vi "subStepper Motor.vi"(8 "error in":errorcluster, 9 "# of Pellet":dbl, 10 "Numeric":dbl, 11 "Arduino Resource":T1={"VISA resource"="", "Board Type"=enum."Uno", "Connection Type"=enum."USB / Serial", "Bytes Per Packet (15)"=15}) -> (0 "error out":errorcluster, 2 "Stepper Step":i32, 3 "Arduino Resource 2":T1={"VISA resource"="", "Board Type"=enum."Uno", "Connection Type"=enum."USB / Serial", "Bytes Per Packet (15)"=15})   [LabVIEW 2016]
uses:
  <vilib>/LabVIEW Interface for Arduino/Type Defs/Arduino Resource.ctl
  <vilib>/LabVIEW Interface for Arduino/Type Defs/Board Type.ctl
  <vilib>/LabVIEW Interface for Arduino/LabVIEW Interface for Arduino.lvlib
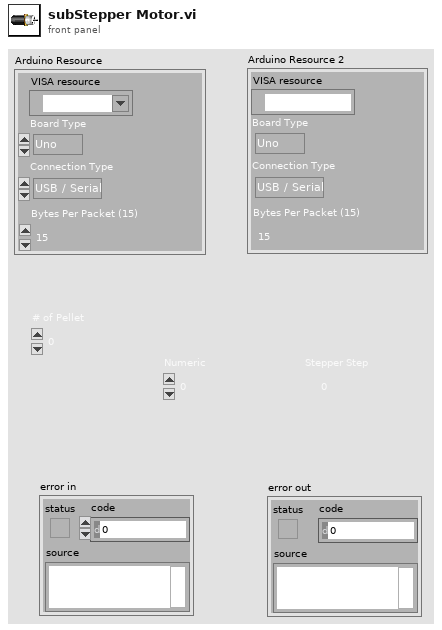
[diagram p1: front panel]
types:
  T1 = typedef "LabVIEW Interface for Arduino.lvlib/Arduino Resource.ctl" = cluster{"VISA resource":refnum<visa-resource-name>, "Board Type":T2, "Connection Type":enum8{"USB / Serial"}, "Bytes Per Packet (15)":u8}
  T2 = typedef "LabVIEW Interface for Arduino.lvlib/Board Type.ctl" = enum16{"Uno", "Dimuelanove w/Atmega 328", "Mega 2560"}
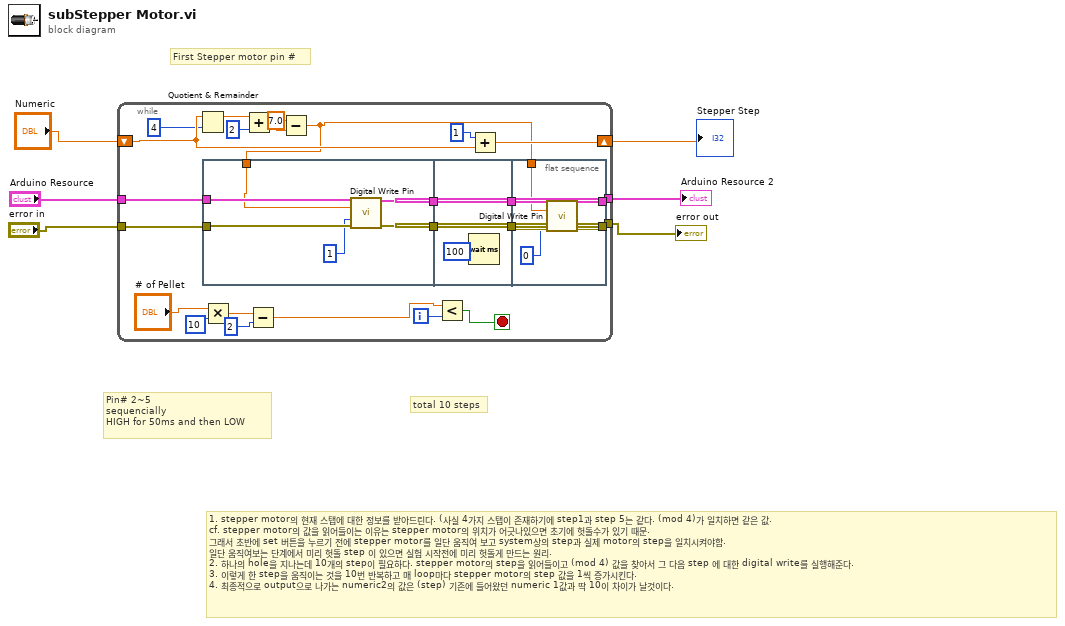
[diagram p0: block diagram]
diagram:
  # "1. stepper motor의 현재 스탭에 대한 정보를 받아드린다. (사실 4가지 스탭이 존재하기에 step1과 step 5는 같다. (mod 4)가 일치하면 같은 값.\ncf. stepper motor의 값을 읽어들이는 이유는 stepper motor의 위치가 어긋나있으면 초기에 헛돌수가 있기 때문. \n그래서 초반에 set 버튼을 누르기 전에 stepper motor를 일단 움직여 보고 system상의 step과 실제 motor의 step을 일치시켜야함.\n일단 움직여보는 단계에서 미리 헛돌 step 이 있으면 실험 시작전에 미리 헛돌게 만드는 원리.\n2. 하나의 hole을 지나는데 10개의 step이 필요하다. stepper motor의 step을 읽어들이고 (mod 4) 값을 찾아서 그 다음 step 에 대한 digital write를 실행해준다.\n3. 이렇게 한 step을 움직이는 것을 10번 반복하고 매 loop마다 stepper motor의 step 값을 1씩 증가시킨다. \n4. 최종적으로 output으로 나가는 numeric2의 값은 (step) 기존에 들어왔던 numeric 1값과 딱 10이 차이가 날것이다."
  # "total 10 steps"
  # "Pin# 2~5\nsequencially\nHIGH for 50ms and then LOW"
  # "First Stepper motor pin #"
  n1 = while {
    tunnel: "Arduino Resource" -> [w30]
    tunnel: "error in" -> [w29]
    shift-right: [w26] -> w1
    shift-left: "Numeric" -> [w18]
    tunnel: [w24] -> w3
    tunnel: [w23] -> w2
    i -> [w28]
    stop <- w27 stop-if-true
    n2 = Quotient & Remainder(x=w18, y=4) -> (x-y*floor(x/y)=w16:dbl)  [unwired: 1 out]
    n3 = flat-sequence {
      tunnel: w30 -> [w36]
      tunnel: w29 -> [w35]
      tunnel: [w34] -> w22
      tunnel: [w33] -> w21
      tunnel: w9 -> [w32]
      tunnel: w22 -> [w39]
      tunnel: w21 -> [w38]
      tunnel: [w39] -> w20
      tunnel: [w38] -> w19
      tunnel: [w43] -> w23
      tunnel: [w44] -> w24
      tunnel: w20 -> [w45]
      tunnel: w19 -> [w42]
      tunnel: w9 -> [w41]
      frame #0 {
        n4 = call <vilib>:"Digital Write Pin.vi"("Arduino Resource"=w36, "Digital I/O Pin (0)"=w32, "Value (0)"=1, "error in"=w35) -> ("Arduino Resource"=w34:T1, "error out"=w33:errorcluster)  [unwired: 10 in]
      }
      frame #1 {
        n5 = Wait (ms)(milliseconds to wait=100) -> ()  [unwired: 1 out]
      }
      frame #2 {
        n6 = call <vilib>:"Digital Write Pin.vi"("Arduino Resource"=w45, "Digital I/O Pin (0)"=w41, "Value (0)"=0, "error in"=w42) -> ("Arduino Resource"=w44:T1, "error out"=w43:errorcluster)  [unwired: 10 in]
      }
    }
    n7 = Multiply(x="# of Pellet", y=10) -> (x*y=w13:dbl)
    n8 = Add(x=w16, y=2) -> (x+y=w8:dbl)
    n9 = Subtract(x=w13, y=2) -> (x-y=w10:dbl)
    n10 = Subtract(x=7.0, y=w8) -> (x-y=w9:dbl)
    n11 = Less?(x=w10, y=w28) -> (x < y?=w27:bool)
    n12 = Add(x=1, y=w18) -> (x+y=w26:dbl)
  }
  "Arduino Resource 2" <- w3
  "error out" <- w2
  "Stepper Step" <- w1
